vi "PulseIn.vi"() -> ()   [LabVIEW 2019]
uses:
  <vilib>/myRIO/Express VI/Onboard IO/DO/DO Express VI.xnode
  <vilib>/myRIO/Instrument Drivers/Onboard IO/DIO/typedefs/DIO Reference.ctl
  <vilib>/myRIO/Instrument Drivers/Onboard IO/DIO/DIO.lvlib
  <vilib>/myRIO/Common/Instrument Driver Framework/myRIO v1.0/DIO/typedefs/DIO Channels List.ctl
  <vilib>/myRIO/Common/Instrument Driver Framework/myRIO v1.0/DIO/typedefs/DIO Channels Enum.ctl
  <vilib>/myRIO/Common/Instrument Driver Framework/Utilities/typedefs/myRIO Generic Hardware Reference.ctl
  <vilib>/myRIO/Common/Instrument Driver Framework/Utilities/typedefs/myRIO v1.0 Reference.ctl
  <vilib>/myRIO/Common/Instrument Driver Framework/Utilities/typedefs/Generic FPGA Reference.ctl
  <vilib>/myRIO/Common/Instrument Driver Framework/Utilities/typedefs/Hardware Version Enum.ctl
  <vilib>/myRIO/Instrument Drivers/Onboard IO/DIO/vis/Write.vi
  <vilib>/myRIO/Instrument Drivers/Onboard IO/DIO/vis/myRIO DIO Open.xnode
  <vilib>/userDefined/High Color/nirio_resource_hc.ctl
  <vilib>/myRIO/Common/Instrument Driver Framework/myRIO v1.0/DIO/vis/myRIO v1.1 Open DIO.vi
  <vilib>/myRIO/Common/Instrument Driver Framework/Utilities/vis/Is FPGA Ref Available.vi
  <vilib>/platform/TimedLoop/XDataNode/XDataNode.xnode
  <vilib>/Platform/TimedLoop/XDataNode/nitl_modes.ctl
  <vilib>/Platform/TimedLoop/XDataNode/XDNodeRunTimeDep.lvlib
  <vilib>/Platform/TimedLoop/XDataNode/wakeup.ctl
  <vilib>/Platform/TimedLoop/XDataNode/timing_clust.ctl
  <instrlib>/Devantech SRF05/Devantech SRF05 PWM (PC).lvlib
  <instrlib>/Devantech CMPS03/driver for PWM/Devantech CMPS03 PWM (PC).lvlib
  <instrlib>/MaxSonar EZ1/driver for PWM/MaxSonar EZ1 PWM (PC).lvlib
panel:
  in  "stop 2":bool
  in  "stop":bool
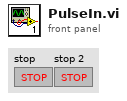
[diagram p1: front panel]
types:
  T1 = typedef "XDNodeRunTimeDep.lvlib/timing_clust.ctl" = cluster{"Expected End [f-1]":u64, "Actual End [f-1]":u64, "Finished Late? [f-1]":bool, "Expected End [i-1]":u64, "Actual End [i-1]":u64, "Finished Late? [i-1]":bool, "Expected Start [i]":u64, "Actual Start [i]":u64, "Expected Start [f]":u64, "Actual Start [f]":u64, "Source Name":string, "Structure Name":string, "Period":i64, "Deadline":i64, "Offset":i64, "Start":i64, "Priority":i32, "Timeout":i32, "Mode":T2, "Wakeup Reason":T3, "Error":errorcluster, "Source Type":string, "Secondary Source Type":string, "Global End Time":u64, "Global Start Time":u64, "Frame Duration":u64, "Iteration Duration":u64, "Assigned CPU":i32, "I/O Scan Engine Mode":u32}
  T2 = typedef "XDNodeRunTimeDep.lvlib/nitl_modes.ctl" = enum32{"No Change", "Process missed periods, maintain original phase", "Discard missed periods, maintain original phase", "Process missed periods, ignore original phase", "Discard missed periods, ignore original phase"}
  T3 = typedef "XDNodeRunTimeDep.lvlib/wakeup.ctl" = enum32{"Normal", "Aborted", "Asynchronous wakeup", "Timing source error", "Timed loop error", "Timeout"}
  T4 = typedef "DIO.lvlib/DIO Reference.ctl" = cluster{"myRIO Reference":T5, "DIO Channels List":T9}
  T5 = typedef "myRIO Generic Hardware Reference.ctl" = cluster{"myRIO Model":T6, "myRIO Hardware Reference":T7}
  T6 = typedef "Hardware Version Enum.ctl" = enum16{"Unknown", "myRIO-1900", "myRIO-1950", "roboRIO", "NI ELVIS RIO CM", "ELVIS III"}
  T7 = typedef "myRIO v1.0 Reference.ctl" = cluster{"Generic FPGA Reference":T8, "Allow multiple opens":bool}
  T8 = typedef "Generic FPGA Reference.ctl" = refnum<k20>
  T9 = typedef "DIO Channels List.ctl" = T10[]
  T10 = typedef "DIO Channels Enum.ctl" = enum16{"Not Connected", "C/DIO0", "C/DIO1", "C/DIO2", "C/DIO3", "C/DIO4", "C/DIO5", "C/DIO6", "C/DIO7", "A/DIO0", "A/DIO1", "A/DIO2", "A/DIO3", "A/DIO4", "A/DIO5", "A/DIO6", "A/DIO7", "A/DIO8", "A/DIO9", "A/DIO10", "A/DIO11", "A/DIO12", "A/DIO13", "A/DIO14", "A/DIO15", "A/DIO16", "A/DIO17", "A/DIO18", "A/DIO19", "B/DIO0", "B/DIO1", "B/DIO2", "B/DIO3", "B/DIO4", "B/DIO5", "B/DIO6", "B/DIO7", "B/DIO8", "B/DIO9", "B/DIO10", "B/DIO11", "B/DIO12", "B/DIO13", "B/DIO14", "B/DIO15", "B/DIO16", "B/DIO17", "B/DIO18", "B/DIO19", "LED0", "LED1", "LED2", "LED3", "Button0", "DIO/DIO0", "DIO/DIO1", "DIO/DIO2", "DIO/DIO3", "DIO/DIO4", "DIO/DIO5", "DIO/DIO6", "DIO/DIO7", "DIO/DIO8", "DIO/DIO9", "SPI/CS0", "SPI/CS1", "SPI/CS2", "SPI/CS3", "LED RADIO (Green)", "LED RADIO (Red)", "LED COMM (Green)", "LED COMM (Red)", "LED MODE (Green)", "LED MODE (Red)"}
  T11 = typedef "nirio_resource_hc.ctl" = tag
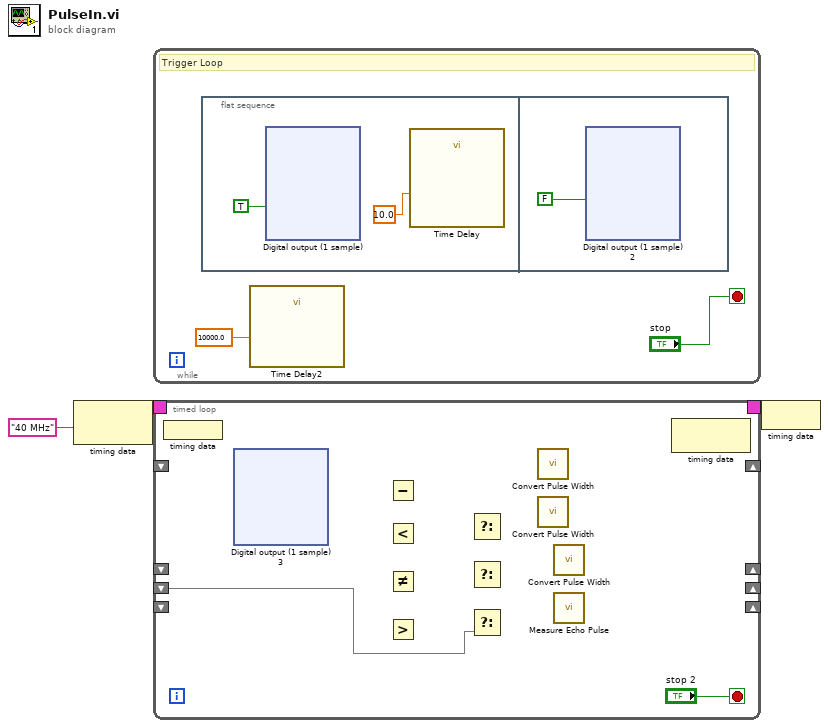
[diagram p0: block diagram]
diagram:
  n1 = node-c288("40 MHz" ("Source Name")) -> (w3:T1)
  n2 = while {
    stop <- "stop" stop-if-true
    # "Trigger Loop"
    n3 = flat-sequence {
      frame #0 {
        n4 = xnode "Digital output (1 sample)"("Trigger (C/DIO1 (DIO1))"=TRUE) -> ()  [unwired: 1 in, 1 out]
        n5 = call "Time Delay"("Delay Time (s)"=10.0) -> ()  [unwired: 10 in, 1 out]
      }
      frame #1 {
        n6 = xnode "Digital output (1 sample) 2"("Trigger (C/DIO1 (DIO1))"=FALSE) -> ()  [unwired: 1 in, 1 out]
      }
    }
    n7 = call "Time Delay2"("Delay Time (s)"=10000.0) -> ()  [unwired: 10 in, 1 out]
  }
  n8 = timed-loop {
    timing: w3 -> [_]
    timing-out: [_] -> w2
    shift-right: _ -> [_]
    shift-left: _ -> [_]
    shift-right: _ -> [_]
    shift-left: _ -> [_]
    shift-right: _ -> [_]
    shift-left: _ -> [w79]
    shift-right: _ -> [_]
    shift-left: _ -> [_]
    stop <- "stop 2" stop-if-true
    n9 = node-c288() -> ()  [unwired: 1 in]
    n10 = xnode "Digital output (1 sample) 3"() -> ()  [unwired: 2 in, 1 out]
    n11 = Subtract() -> ()  [unwired: 2 in, 1 out]
    n12 = Less?() -> ()  [unwired: 2 in, 1 out]
    n13 = Not Equal?() -> ()  [unwired: 2 in, 1 out]
    n14 = Greater?() -> ()  [unwired: 2 in, 1 out]
    n15 = Select() -> ()  [unwired: 3 in, 1 out]
    n16 = Select() -> ()  [unwired: 3 in, 1 out]
    n17 = Select(f=w79) -> ()  [unwired: 2 in, 1 out]
    n18 = call <instrlib>:"Convert Pulse Width.vi"() -> ()  [unwired: 11 in, 1 out]
    n19 = call <instrlib>:"Convert Pulse Width.vi"() -> ()  [unwired: 11 in, 1 out]
    n20 = call <instrlib>:"Convert Pulse Width.vi"() -> ()  [unwired: 11 in, 1 out]
    n21 = call <instrlib>:"Measure Echo Pulse.vi"() -> ()  [unwired: 8 in, 4 out]
    n22 = node-c288() -> ()  [unwired: 1 in, 1 out]
  }
  n23 = node-c288(w2) -> ()
